vi "Res Mirror um to Volts.vi"(1 "Image Size (um)":dbl) -> (0 "Voltage (V)":dbl)   [LabVIEW 2014]
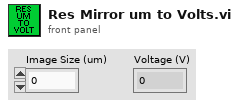
[diagram p1: front panel]
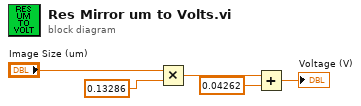
[diagram p0: block diagram]
diagram:
  n1 = Multiply(x="Image Size (um)", y=0.13286) -> (x*y=w4:dbl)
  n2 = Add(x=w4, y=0.04262) -> (x+y=→"Voltage (V)":dbl)
